vi "TS Initialize.vi"(6 "Cluster":T1, 8 "error in":errorcluster, 10 "Device \n(Case Sensitive)":string="Report", 11 "Application Directory":path) -> (0 "error out":errorcluster, 3 "Report out":refnum<class "Report.lvclass">)   [LabVIEW 2019]
uses:
  Report.lvclass
  PPL/Instruments.lvlibp/Instruments.lvclass
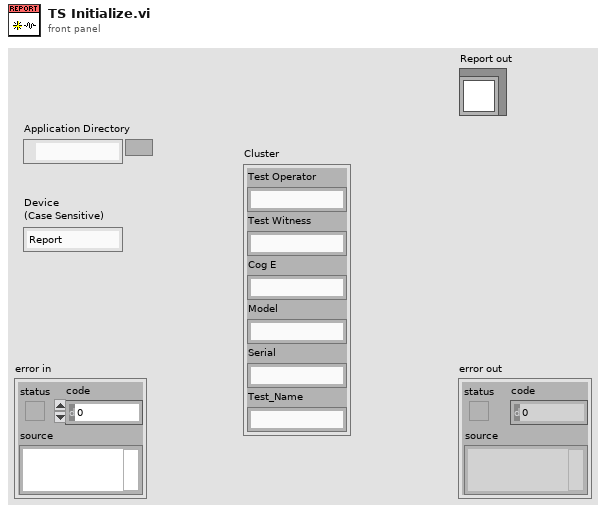
[diagram p1: front panel]
types:
  T1 = cluster{"Test Operator":string, "Test Witness":string, "Cog E":string, "Model":string, "Serial":string, "Test_Name":string}
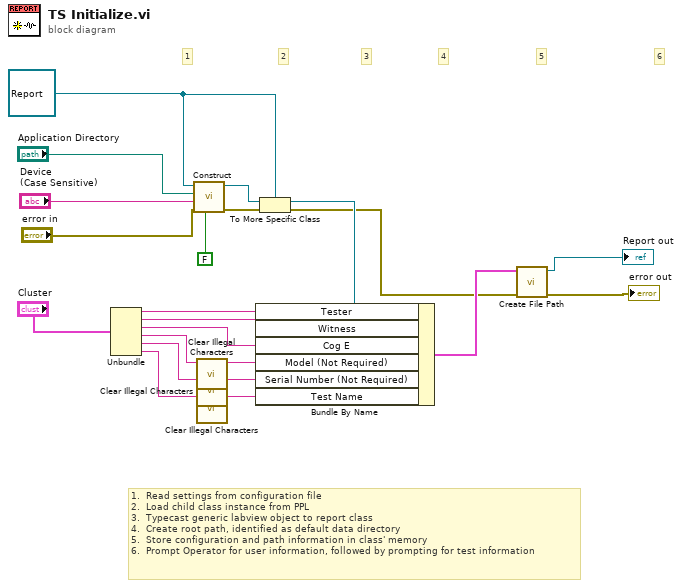
[diagram p0: block diagram]
diagram:
  w21 = refnum<class "Report.lvclass"> refnum ("Report in")
  # "6"
  # "5"
  # "4"
  # "1.  Read settings from configuration file\n2.  Load child class instance from PPL\n3.  Typecast generic labview object to report class\n4.  Create root path, identified as default data directory\n5.  Store configuration and path information in class' memory\n6.  Prompt Operator for user information, followed by prompting for test information"
  # "3"
  # "2"
  # "1"
  n1 = Unbundle("Cluster") -> ("Test Operator"=w13:string, "Test Witness"=w12:string, "Cog E"=w11:string, "Model"=w6:string, "Serial"=w5:string, "Test_Name"=w2:string)
  n2 = call "Construct.vi"("Scripting"=FALSE, "error in (no error)"="error in", "Handle"="Device \n(Case Sensitive)", "Application Directory"="Application Directory", "Instruments in"=w21) -> ("error out"=w20:errorcluster, "Instruments out"=w22:refnum<class "Instruments.lvclass">)  [unwired: 5 in]
  n3 = call "Clear Illegal Characters.vi"("String in"=w6) -> ("Safe String out"=w4:string)  [unwired: 10 in]
  n4 = call "Clear Illegal Characters.vi"("String in"=w5) -> ("Safe String out"=w3:string)  [unwired: 10 in]
  n5 = call "Clear Illegal Characters.vi"("String in"=w2) -> ("Safe String out"=w1:string)  [unwired: 10 in]
  n6 = To More Specific Class(target class=w21, reference=w22, error in=w20) -> (specific class reference=w15:refnum<class "Report.lvclass">, error out=w9:errorcluster)
  n7 = Bundle By Name(cluster=w15, "Tester"=w13, "Witness"=w12, "Cog E"=w11, "Model (Not Required)"=w4, "Serial Number (Not Required)"=w3, "Test Name"=w1) -> (w10:cluster{})
  n8 = call "Create File Path.vi"("error in"=w9, "Report in"=w10) -> ("error out"=→"error out":errorcluster, "Report out"=→"Report out":refnum<class "Report.lvclass">)  [unwired: 8 in]
